vi "Fit VI window to Largest Dec.vi"(4 "error in (no error)":errorcluster, 6 "border spacing (2 px)":i32=2, 7 "VI Ref (calling VI)":refnum<vi>) -> (0 "error out":errorcluster, 3 "dup VI Ref":refnum<vi>)   [LabVIEW 2011]
doc: "This utility will fit (resize and center) a VI (defined by the \"VI Ref\" input) about the largest decoration in that VI. It will add a border defined by border spacing in units of pixels. If there are no decorations found in the VI it is a no-op and will not produce an error. Unfortunately, this VI can not find locked decorations (yet)."
panel:
  # "[OpenG VI Tags] ***Do Not Remove***\nCVS Revision = 1.3\nCVS Revision Date = Sat Nov  6 20:04:09 2004\nPackage = oglib_appcontrol-2.7-1\nDepends ="
  # "Fit VI window to Largest Decoration.vi - Fits a VI's front panel window\nto its largest decoration size.\n\nCopyright (C) 2002 James Kring jim@jimkring.com\nCopyright (C) 2002 Cal-Bay Systems, Inc. info@calbay.com\n\nPlease visit http://www.OpenG.org to learn about the\nOpen Source LabVIEW software movement.\n\nThis library is free software; you can redistribute it and/or\nmodify it under the terms of the GNU Lesser General Public\nLicense as published by the Free Software Foundation; either\nversion 2.1 of the License, or (at your option) any later version.\nThis library is distributed in the hope that it will be useful,\nbut WITHOUT ANY WARRANTY; without even the implied warranty of\nMERCHANTABILITY or FITNESS FOR A PARTICULAR PURPOSE. See the GNU\nLesser General Public License for more details.\nYou should have received a copy of the GNU Lesser General Public\nLicense along with this library; if not, write to the Free Software\nFoundation, Inc., 59 Temple Place, Suite 330, Boston, MA 02111-1307 USA"
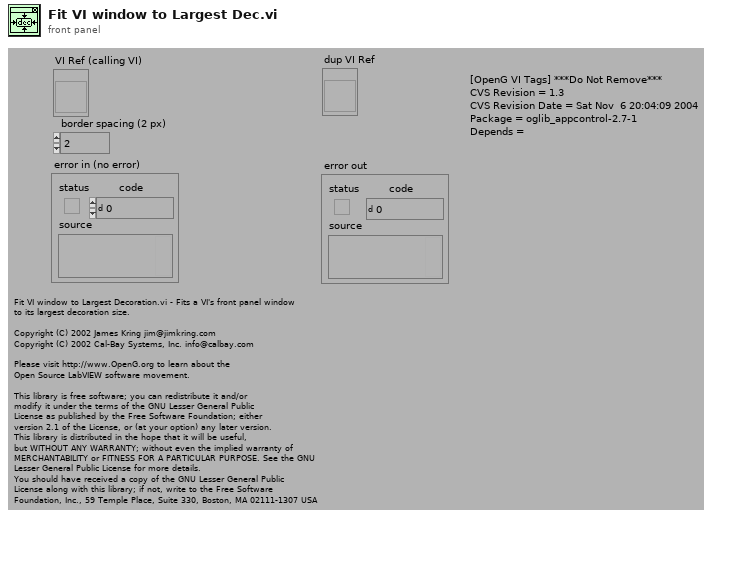
[diagram p1: front panel]
types:
  T1 = typedef "LVRectTypeDef.ctl" = cluster{"left":i16, "top":i16, "right":i16, "bottom":i16}
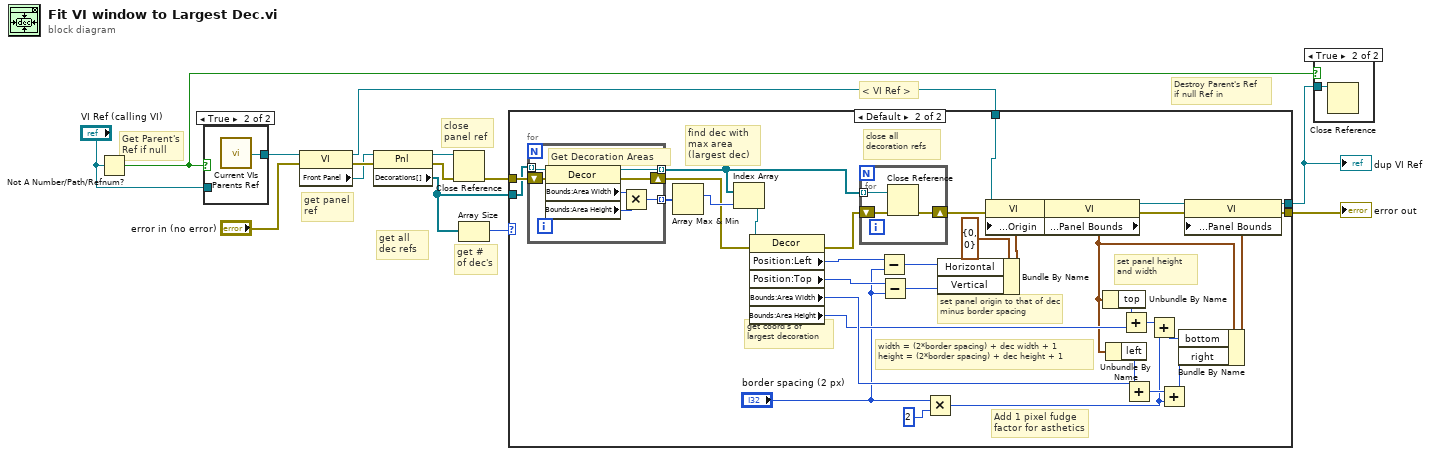
[diagram p0: block diagram]
diagram:
  # "Destroy Parent's Ref\nif null Ref in"
  # "Get Parent's\nRef if null"
  # "get # of dec's"
  # "get panel ref"
  # "get all dec refs"
  # "close panel ref"
  # "< VI Ref >"
  n1 = Not A Number/Path/Refnum?(number/path/refnum="VI Ref (calling VI)") -> (NaN/Path/Refnum?=w2:bool)
  n2 = case shown="True" w2 {
    tunnel: [w15 w16] -> w3
    tunnel: "VI Ref (calling VI)" -> [w15 _]
    frame False {
    }
    frame True {
      n3 = call "Current VIs Parents Ref.vi"() -> ("Calling VI's reference"=w16:refnum<vi>)  [unwired: 2 in]
    }
  }
  n4 = property on="Property Node" class="VI"(reference=w3, error in="error in (no error)") -> (reference out=w14:refnum<vi>, error out=w12:errorcluster, "Front Panel"=w9:refnum<vi>)
  n5 = property on="Property Node" class="Pnl"(reference=w9, error in=w12) -> (reference out=w13:refnum<vi>, error out=w11:errorcluster, "Decorations[]"=w6:refnum<vi>[])
  n6 = Close Reference(reference=w13, error in (no error)=w11) -> (error out=w8:errorcluster)
  n7 = Array Size(array=w6) -> (size(s)=w5:i32)
  n8 = case shown="Default" w5 {
    tunnel: w14 -> [w18 w51]
    tunnel: w8 -> [w17 w34]
    tunnel: [w17 w22] -> w7
    tunnel: [w18 w21] -> w1
    tunnel: w6 -> [_ w20]
    frame 0 {
      # "do nothing if no decorations"
    }
    frame Default {
      # "width = (2*border spacing) + dec width + 1\nheight = (2*border spacing) + dec height + 1"
      # "set panel height and width"
      # "set panel origin to that of dec minus border spacing"
      # "close all  decoration refs"
      # "get coord's of largest decoration"
      # "Add 1 pixel fudge factor for asthetics"
      # "find dec with max area (largest dec)"
      n9 = for {
        tunnel: w20 -> [w60] mode=indexing
        tunnel: [w57] -> w33 mode=indexing
        shift-right: [w55] -> w29
        shift-left: w34 -> [w56]
        tunnel: [w54] -> w31 mode=indexing
        # "Get Decoration Areas"
        n10 = property class="Decor"(reference=w60, error in=w56) -> (reference out=w54:refnum<vi>, error out=w55:errorcluster, "Bounds:Area Width"=w59:u32, "Bounds:Area Height"=w58:u32)
        n11 = Multiply(x=w59, y=w58) -> (x*y=w57:u32)
      }
      n12 = Array Max & Min(array=w33) -> (max index (indices)=w32:i32)  [unwired: 3 out]
      n13 = Index Array(array=w31, index=w32) -> (element=w30:refnum<vi>)
      n14 = property class="Decor"(reference=w30, error in=w29) -> (error out=w28:errorcluster, "Position:Left"=w37:i32, "Position:Top"=w40:i32, "Bounds:Area Width"=w45:u32, "Bounds:Area Height"=w43:u32)  [unwired: 1 out]
      n15 = for {
        tunnel: w31 -> [w63] mode=indexing
        shift-right: [w61] -> w25
        shift-left: w28 -> [w62]
        n16 = Close Reference(reference=w63, error in (no error)=w62) -> (error out=w61:errorcluster)
      }
      n17 = Subtract(x=w37, y="border spacing (2 px)") -> (x-y=w38:i32)
      n18 = Subtract(x=w40, y="border spacing (2 px)") -> (x-y=w39:i32)
      n19 = Multiply(x="border spacing (2 px)", y=u32 2) -> (x*y=w19:u32)
      n20 = Bundle By Name(cluster=cluster{"Horizontal":i16, "Vertical":i16} {"Horizontal"=0, "Vertical"=0} ("Front Panel Window:Origin"), "Horizontal"=w38, "Vertical"=w39) -> (w35:cluster{"Horizontal":i16, "Vertical":i16})
      n21 = property on="Property Node" class="VI"(reference=w51, error in=w25, "Front Panel Window:Origin"=w35) -> (reference out=w52:refnum<vi>, error out=w24:errorcluster)
      n22 = property on="Property Node" class="VI"(reference=w52, error in=w24) -> (reference out=w53:refnum<vi>, error out=w23:errorcluster, "Front Panel Window:Panel Bounds"=w41:T1)
      n23 = Unbundle By Name(w41) -> ("top"=w42:i16)
      n24 = Unbundle By Name(w41) -> ("left"=w44:i16)
      n25 = Add(x=w42, y=w43) -> (x+y=w49:u32)
      n26 = Add(x=w44, y=w45) -> (x+y=w47:u32)
      n27 = Add(x=w49, y=w19) -> (x+y=w50:u32)
      n28 = Add(x=w47, y=w19) -> (x+y=w48:u32)
      n29 = Bundle By Name(cluster=w41, "bottom"=w50, "right"=w48) -> (w46:T1)
      n30 = property on="Property Node" class="VI"(reference=w53, error in=w23, "Front Panel Window:Panel Bounds"=w46) -> (reference out=w21:refnum<vi>, error out=w22:errorcluster)
    }
  }
  "error out" <- w7
  "dup VI Ref" <- w1
  n31 = case shown="True" w2 {
    tunnel: w1 -> [_ w64]
    frame False {
    }
    frame True {
      n32 = Close Reference(reference=w64) -> ()  [unwired: 1 in, 1 out]
    }
  }
